vi "metadata_to_textArray.vi"(11 "metadata to save":T1 {"cell stats"."STD" format="%010.2f"; "cell stats"."Variance" format="%010.2f"; "cell stats"."Rt (MOhms)" format="%010.2f"; "cell stats"."tau (ms)" format="%08.2g"; "cell stats"."Cm (pF)" format="%08.2f"; "cell stats"."Ra (MOhms)" format="%010.2f"; "cell stats"."Rm (MOhms)" format="%010.2f"; "cell stats"."Ihold (pA)" format="%010.2f"}) -> (3 "xml string out":string)   [LabVIEW 2019]
uses:
  Controls/metadata_to_save.ctl
  Controls/cell_stats-v02.ctl
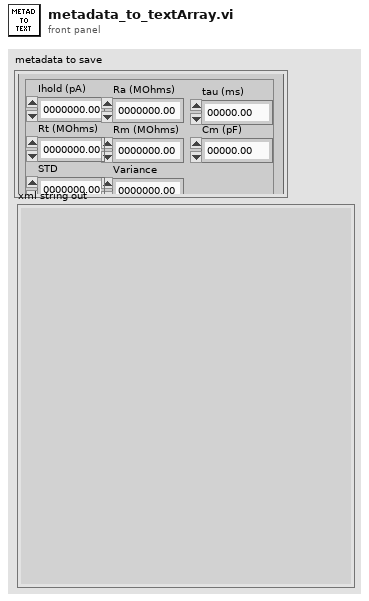
[diagram p1: front panel]
types:
  T1 = typedef "metadata_to_save.ctl" = cluster{"cell stats":T2}
  T2 = typedef "cell_stats-v02.ctl" = cluster{"Ihold (pA)":dbl, "Rm (MOhms)":dbl, "Ra (MOhms)":dbl, "Cm (pF)":dbl, "tau (ms)":dbl, "Rt (MOhms)":dbl, "Variance":dbl, "STD":dbl}
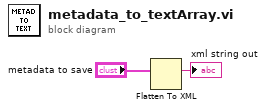
[diagram p0: block diagram]
diagram:
  n1 = Flatten To XML(anything="metadata to save") -> (xml string=→"xml string out":string)
